vi "KepcoDCPwr Configure Output Enabled.vi"(0 "VISA Session":refnum<visa-resource-name>, 5 "Model In":string, 9 "Input enabled (True)":bool=TRUE, 11 "error in (no error)":errorcluster {"code" format="%.0x"}) -> (4 "VISA Session Out":refnum<visa-resource-name>, 6 "Model Out":string, 15 "error out":errorcluster {"code" format="%.0x"})   [LabVIEW 2020]
doc: "Configures whether the signal that the power supply produces on a channel appears at the output connector."
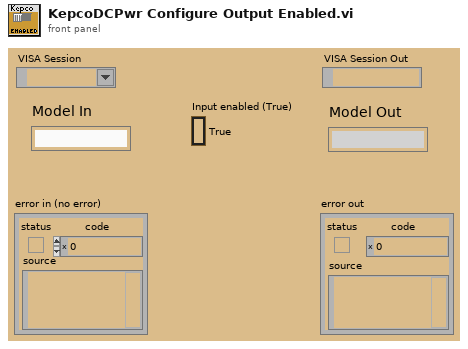
[diagram p1: front panel]
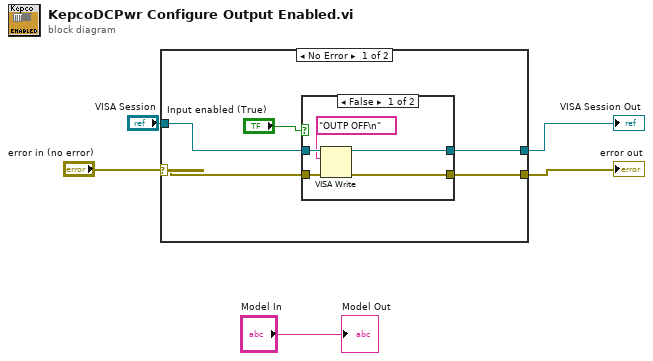
[diagram p0: block diagram]
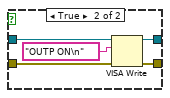
[diagram p2: hidden frame]
diagram:
  n1 = case shown="No Error" "error in (no error)" {
    selector: "error in (no error)" -> [w8 w21]
    tunnel: "VISA Session" -> [w9 w22]
    tunnel: [w7 w21] -> w3
    tunnel: [w6 w22] -> w2
    frame No Error {
      n2 = case shown="False" "Input enabled (True)" {
        tunnel: [w14 w19] -> w6
        tunnel: [w12 w18] -> w7
        tunnel: w8 -> [w13 w17]
        tunnel: w9 -> [w15 w16]
        frame False {
          n3 = VISA Write(VISA resource name=w15, write buffer="OUTP OFF\n", error in (no error)=w13) -> (VISA resource name out=w14:refnum<visa-resource-name>, error out=w12:errorcluster)  [unwired: 1 out]
        }
        frame True {
          n4 = VISA Write(VISA resource name=w16, write buffer="OUTP ON\n", error in (no error)=w17) -> (VISA resource name out=w19:refnum<visa-resource-name>, error out=w18:errorcluster)  [unwired: 1 out]
        }
      }
    }
    frame Error {
    }
  }
  "error out" <- w3
  "VISA Session Out" <- w2
  "Model Out" <- "Model In"
